vi "Read.vi"(2 "niInstr AXI4-Stream Reader v1 FPGA in":refnum<class "niInstr AXI4-Stream Reader v1 FPGA.lvclass">, 12 "ready for output":bool) -> (3 "tlast":bool, 4 "tdata":bool[](array[boolean]), 6 "tstrb":bool[](array[boolean]), 8 "tkeep":bool[](array[boolean]), 10 "output valid":bool, 14 "tuser":bool[](array[boolean]))   [LabVIEW 2015, in "niInstr AXI4-Stream Reader v1 FPGA.lvclass"]
doc: "Performs a read operation on the AXI4-Stream Reader.\n\n<B>Input Parameters</B>\n\n<B>niInstr AXI4-Stream Reader v1 FPGA in</B> takes in a reference to the AXI4-Stream Reader from the previous VI\n\n<B>ready for output</B> specifies whether the AXI4-Stream Reader is ready to transmit data.\n\n<B>Output Parameters</B>\n\n<B>tlast</B> is the TLAST signal for the AXI4-Stream Reader.\n\n<B>tdata</B> is the TDATA signal for the AXI4-Stream Reader.\n\n<B>tstrb</B> is the TSTRB signal for the AXI4-Stream Reader.\n\n<B>tkeep</B> is the TKEEP signal for the AXI4-Stream Reader.\n\n<B>output valid</B> is true when the output is valid.\n\n<B>tuser</B> is the TUSER signal for the AXI4-Stream Reader."
uses:
  <instrlib>/_niInstr/CLIP Adapters/v1/FPGA/AXI4-Stream/Reader/niInstr AXI4-Stream Reader v1 FPGA.lvclass
  <instrlib>/_niInstr/CLIP Adapters/v1/FPGA/AXI4-Stream/Reader/niInstr AXI4-Stream Reader v1 FPGA.lvclass/niInstr AXI4-Stream Reader v1 FPGA.ctl
  <vilib>/rvi/eio/common/nirviEmuTemplateMethod_errors.vi
  <vilib>/eio/EIONode/EIONode.xnode
  <instrlib>/_niInstr/Basic Elements/v1/FPGA/niInstr Basic Elements v1 FPGA.lvlib
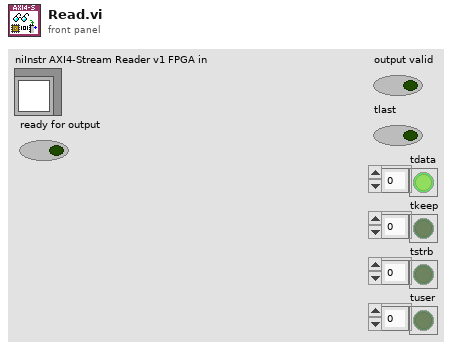
[diagram p1: front panel]
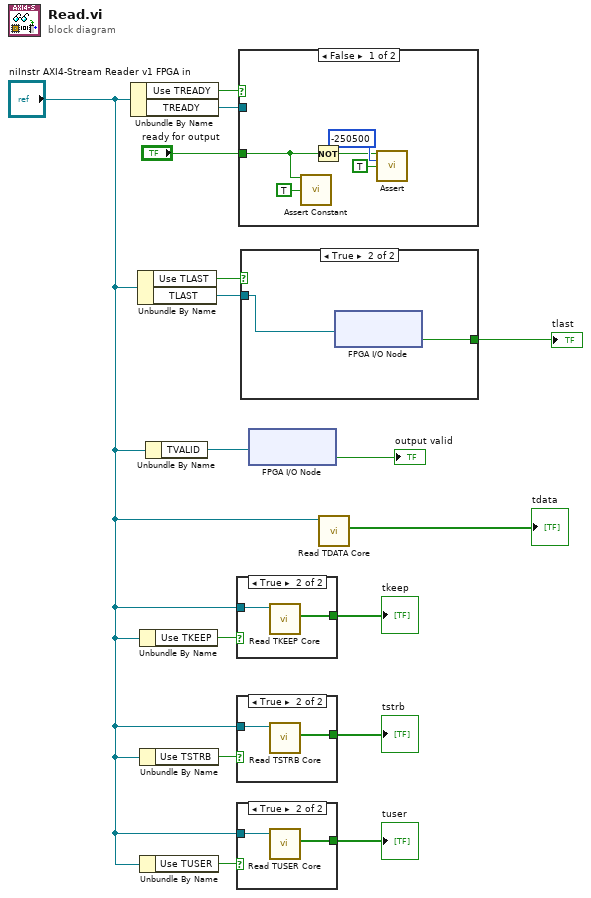
[diagram p0: block diagram]
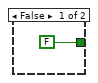
[diagram p5: hidden frame]
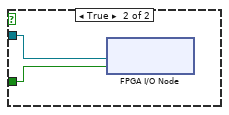
[diagram p6: hidden frame]
diagram:
  n1 = Unbundle By Name("niInstr AXI4-Stream Reader v1 FPGA in") -> ("Use TREADY"=w16:bool, "TREADY"=w15:refnum<k21>)
  n2 = Unbundle By Name("niInstr AXI4-Stream Reader v1 FPGA in") -> ("Use TLAST"=w13:bool, "TLAST"=w12:refnum<k21>)
  n3 = Unbundle By Name("niInstr AXI4-Stream Reader v1 FPGA in") -> ("Use TKEEP"=w7:bool)
  n4 = Unbundle By Name("niInstr AXI4-Stream Reader v1 FPGA in") -> ("Use TSTRB"=w5:bool)
  n5 = Unbundle By Name("niInstr AXI4-Stream Reader v1 FPGA in") -> ("Use TUSER"=w3:bool)
  n6 = Unbundle By Name("niInstr AXI4-Stream Reader v1 FPGA in") -> ("TVALID"=w10:refnum<k21>)
  n7 = case shown="True" w7 {
    tunnel: "niInstr AXI4-Stream Reader v1 FPGA in" -> [_ w18]
    tunnel: [_ w17] -> w6
    frame False {
    }
    frame True {
      n8 = call-dynamic "Read TKEEP Core.vi"("niInstr AXI4-Stream Reader v1 FPGA in"=w18) -> ("value"=w17:bool[])  [unwired: 9 in, 1 out]
    }
  }
  "tkeep" <- w6
  n9 = case shown="True" w5 {
    tunnel: "niInstr AXI4-Stream Reader v1 FPGA in" -> [_ w20]
    tunnel: [_ w19] -> w4
    frame False {
    }
    frame True {
      n10 = call-dynamic "Read TSTRB Core.vi"("niInstr AXI4-Stream Reader v1 FPGA in"=w20) -> ("value"=w19:bool[])  [unwired: 9 in, 1 out]
    }
  }
  "tstrb" <- w4
  n11 = case shown="True" w3 {
    tunnel: "niInstr AXI4-Stream Reader v1 FPGA in" -> [_ w22]
    tunnel: [_ w21] -> w1
    frame False {
    }
    frame True {
      n12 = call-dynamic "Read TUSER Core.vi"("niInstr AXI4-Stream Reader v1 FPGA in"=w22) -> ("value"=w21:bool[])  [unwired: 9 in, 1 out]
    }
  }
  "tuser" <- w1
  n13 = case shown="False" w16 {
    tunnel: w15 -> [_ w29]
    tunnel: "ready for output" -> [w26 w28]
    frame False {
      n14 = call <instrlib>:"Assert Constant.vi"("constant terminal"=w26, "enable show error"=TRUE) -> ()  [unwired: 14 in]
      n15 = Not(x=w26) -> (.not. x?=w23:bool)
      n16 = call <instrlib>:"Assert.vi"("assert"=w23, "error code"=-250500, "enable show error"=TRUE) -> ()  [unwired: 13 in]
    }
    frame True {
      n17 = xnode "FPGA I/O Node"("I/O Item"=w28, "FPGA I/O In"=w29) -> ()  [unwired: 1 out]
    }
  }
  n18 = case shown="True" w13 {
    tunnel: w12 -> [_ w32]
    tunnel: [FALSE ("I/O Item") w31] -> w11
    frame False {
    }
    frame True {
      n19 = xnode "FPGA I/O Node"("FPGA I/O In"=w32) -> ("I/O Item"=w31:bool)  [unwired: 1 out]
    }
  }
  "tlast" <- w11
  n20 = xnode "FPGA I/O Node"("FPGA I/O In"=w10) -> ("I/O Item"=→"output valid":bool)  [unwired: 1 out]
  n21 = call-dynamic "Read TDATA Core.vi"("niInstr AXI4-Stream Reader v1 FPGA in"="niInstr AXI4-Stream Reader v1 FPGA in") -> ("tdata value"=→"tdata":bool[])  [unwired: 9 in, 1 out]
